vi "To String.vi"(8 "error in (no error)":errorcluster, 11 "File Path Result in":refnum<class "File Path Result.lvclass">) -> (0 "error out":errorcluster, 2 "String":string, 3 "File Path Result out":refnum<class "File Path Result.lvclass">)   [LabVIEW 2016, in "File Path Result.lvclass"]
uses:
  File Path Result.lvclass
  Acquired Result/Acquired Result.lvclass
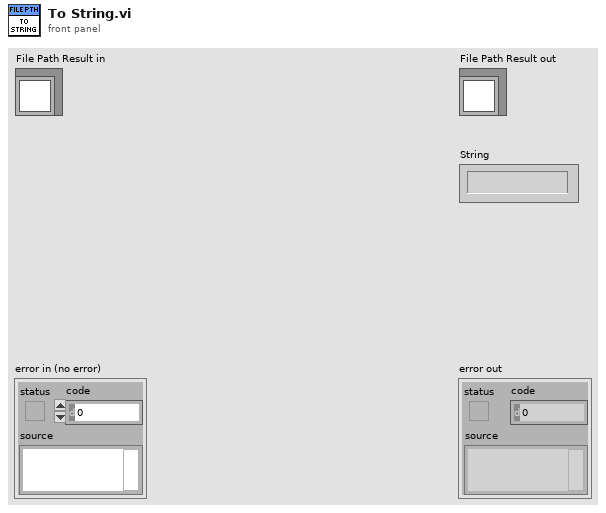
[diagram p1: front panel]
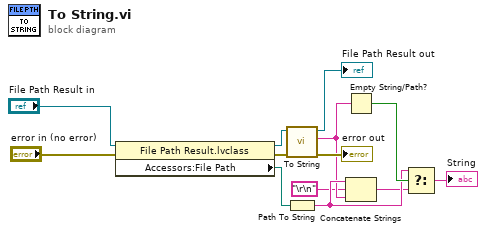
[diagram p0: block diagram]
diagram:
  n1 = property class="File Path Result.lvclass"(reference="File Path Result in", error in="error in (no error)") -> (reference out=w8:refnum<class "File Path Result.lvclass">, error out=w12:errorcluster, "Accessors:File Path"=w10:path)
  n2 = call-parent "To String.vi"("error in (no error)"=w12, "Acquired Result in"=w8) -> ("error out"=→"error out":errorcluster, "String"=w3:string, "Acquired Result out"=→"File Path Result out":refnum<class "File Path Result.lvclass">)  [unwired: 7 in]
  n3 = Path To String(path=w10) -> (string=w4:string)
  n4 = Empty String/Path?(string/path=w3) -> (empty?=w6:bool)
  n5 = Concatenate Strings(w4, "\r\n", w3) -> (w1:string)
  n6 = Select(t=w4, s=w6, f=w1) -> (s? t:f=→"String":string)
